vi "HEWH Read Power.vi"(0 "VISA resource name":refnum<visa-resource-name>="WT500", 11 "error in (no error)":errorcluster) -> (3 "PowerClass":T2={"Off"=FALSE, "On"=TRUE, "Logic"=FALSE, "Compressor"=FALSE, "1Heater"=TRUE, "1Heat+Comp"=FALSE, "2Heaters"=FALSE, "2Heat+Comp"=FALSE, "Fault-OverPwr"=FALSE}, 4 "VISA resource name out":refnum<visa-resource-name>="WT500", 6 "PowerData":T1={"Voltage"=236.2, "Current"=17.749, "Power"=4192.0, "WattHours"=0.0}, 15 "error out":errorcluster)   [LabVIEW 2009]
uses:
  PowerClassification.ctl
panel:
  out "CycleCount":dbl
  in  "Local?":bool
  in  "I Range (7: 40A)":u16(ring)=6 items=["AUTO", "500 mA", "1 A", "2 A", "5 A", "10 A", "20 A", "40 A", "S-AUTO", "50 mV", "100 mV", "200 mV", "500 mV", "1 V", "2 V", "5 V", "10 V", "250 mA", "500 mA", "1 A", "2.5 A", "5 A", "10 A", "20 A", "25 mV", "50 mV", "100 mV", "250 mV", "500 mV", "1 V", "2.5 V", "5 V"]
  in  "V Range (8: 1000V)":u16(ring)=6 items=["AUTO", "15", "30", "60", "100", "150", "300", "600", "1000", "7.5", "15", "30", "50", "75", "150", "300", "500"]
  in  "Logic":dbl=5.0
  in  "Fault Limit":dbl=5000.0
  in  "Heating Element":dbl=4300.0
  in  "Compressor":dbl=550.0
  in  "Off Limit":dbl=0.5
  out "Scan Error":bool
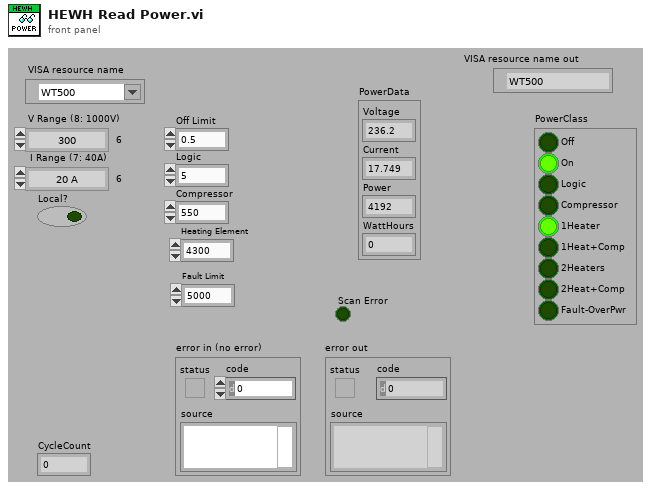
[diagram p1: front panel]
types:
  T1 = cluster{"Voltage":dbl, "Current":dbl, "Power":dbl, "WattHours":dbl}
  T2 = typedef "PowerClassification.ctl" = cluster{"Off":bool, "On":bool, "Logic":bool, "Compressor":bool, "1Heater":bool, "1Heat+Comp":bool, "2Heaters":bool, "2Heat+Comp":bool, "Fault-OverPwr":bool}
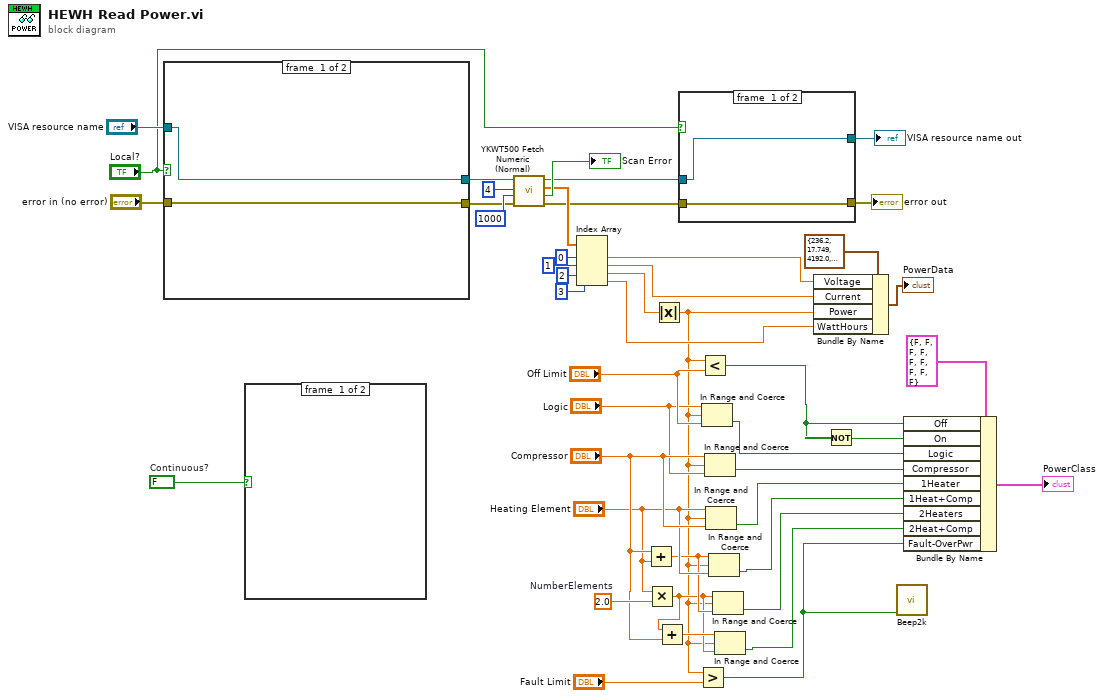
[diagram p0: block diagram]
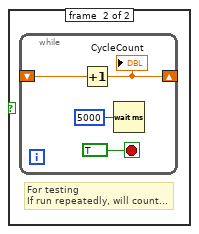
[diagram p2: hidden frame]
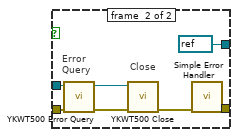
[diagram p3: hidden frame]
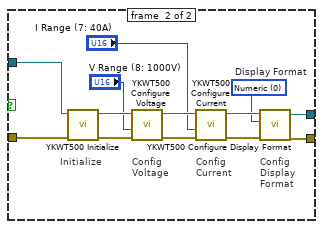
[diagram p4: hidden frame]
diagram:
  w8 = FALSE  # Continuous?
  w36 = 2.0  # NumberElements
  n1 = case shown="True" "Local?" {
    tunnel: "error in (no error)" -> [w46 w51]
    tunnel: "VISA resource name" -> [w47 w50]
    tunnel: [w46 w49] -> w17
    tunnel: [w47 w48] -> w16
    frame #0 {
    }
    frame #1 {
      w52 = u16 0 items=["Numeric", "Wave", "Bar", "Vector", "Trend"]  # Display Format
      # "Config\nDisplay\nFormat"
      # "Config\nCurrent"
      # "Config\nVoltage"
      # "Initialize"
      n2 = call <instrlib>:"YKWT500 Initialize.vi"("error in (no error)"=w51, "VISA resource name"=w50) -> ("error out"=w60:errorcluster, "VISA resource name out"=w58:refnum<visa-resource-name>)  [unwired: 8 in]
      n3 = call <instrlib>:"YKWT500 Configure Voltage.vi"("error in (no error)"=w60, "Voltage Range (8: 1000V)"="V Range (8: 1000V)", "VISA resource name"=w58) -> ("error out"=w59:errorcluster, "VISA resource name out"=w57:refnum<visa-resource-name>)  [unwired: 7 in]
      n4 = call <instrlib>:"YKWT500 Configure Current.vi"("error in (no error)"=w59, "Current Range (7: 40A)"="I Range (7: 40A)", "VISA resource name"=w57) -> ("error out"=w53:errorcluster, "VISA resource name out"=w54:refnum<visa-resource-name>)  [unwired: 7 in]
      n5 = call <instrlib>:"YKWT500 Configure Display Format.vi"("error in (no error)"=w53, "Display Format (0: Numeric)"=w52, "VISA resource name"=w54) -> ("error out"=w49:errorcluster, "VISA resource name out"=w48:refnum<visa-resource-name>)  [unwired: 7 in]
    }
  }
  n6 = case shown="True" w8 {
    frame #0 {
    }
    frame #1 {
      # "For testing\nIf run repeatedly, will count..."
      n7 = while {
        shift-right: [w63] -> _
        shift-left: _ -> [w62]
        stop <- TRUE stop-if-true
        n8 = Increment(x=w62) -> (x+1=w63:dbl)
        "CycleCount" <- w63
        n9 = Wait (ms)(milliseconds to wait=u32 5000) -> ()  [unwired: 1 out]
      }
    }
  }
  n10 = call <instrlib>:"YKWT500 Fetch Numeric (Normal).vi"("error in (no error)"=w17, "Timeout (10000 ms)"=u32 1000, "Number of Item (255)"=4, "VISA resource name"=w16) -> ("error out"=w15:errorcluster, "Scan Error"=→"Scan Error":bool, "Measurement Value"=w42:dbl[], "VISA resource name out"=w13:refnum<visa-resource-name>)  [unwired: 4 in]
  n11 = Index Array(array=w42, index #1=0 ("index"), index #2=1 ("index"), index #3=2 ("index"), index #4=3 ("index")) -> (element #1=w1:dbl, element #2=w2:dbl, element #3=w38:dbl, element #4=w4:dbl)
  n12 = Add(x="Compressor", y="Heating Element") -> (x+y=w21:dbl)
  n13 = Multiply(x="Heating Element", y=w36) -> (x*y=w20:dbl)
  n14 = Absolute Value(x=w38) -> (abs(x)=w3:dbl)
  n15 = Add(x=w20, y="Compressor") -> (x+y=w34:dbl)
  n16 = case shown="True" "Local?" {
    tunnel: w15 -> [w65 w70]
    tunnel: [w65 w69] -> w14
    tunnel: w13 -> [w66 w68]
    tunnel: [w66 refnum<visa-resource-name> refnum ("VISA resource name out")] -> w11
    frame #0 {
    }
    frame #1 {
      # "Error\nQuery"
      # "Close"
      n17 = call <instrlib>:"YKWT500 Error Query.vi"("error in (no error)"=w70, "VISA resource name"=w68) -> ("error out"=w72:errorcluster, "VISA resource name out"=w71:refnum<visa-resource-name>)  [unwired: 6 in, 2 out]
      n18 = call <instrlib>:"YKWT500 Close.vi"("error in (no error)"=w72, "VISA resource name"=w71) -> ("error out"=w73:errorcluster)  [unwired: 9 in]
      n19 = call <vilib>:"Simple Error Handler.vi"("error in (no error)"=w73) -> ("error out"=w69:errorcluster)  [unwired: 4 in, 4 out]
    }
  }
  "error out" <- w14
  "VISA resource name out" <- w11
  n20 = Greater?(x=w3, y="Fault Limit") -> (0:w9:bool)
  n21 = Less?(x=w3, y="Off Limit") -> (x < y?=w31:bool)
  n22 = In Range and Coerce(upper limit="Logic", x=w3, lower limit="Off Limit") -> (In Range?=w29:bool)  [unwired: 1 out]
  n23 = In Range and Coerce(upper limit="Compressor", x=w3, lower limit="Logic") -> (In Range?=w28:bool)  [unwired: 1 out]
  n24 = In Range and Coerce(upper limit="Heating Element", x=w3, lower limit="Compressor") -> (In Range?=w27:bool)  [unwired: 1 out]
  n25 = In Range and Coerce(upper limit=w21, x=w3, lower limit="Heating Element") -> (In Range?=w26:bool)  [unwired: 1 out]
  n26 = In Range and Coerce(upper limit=w20, x=w3, lower limit=w21) -> (In Range?=w25:bool)  [unwired: 1 out]
  n27 = In Range and Coerce(upper limit=w34, x=w3, lower limit=w20) -> (In Range?=w24:bool)  [unwired: 1 out]
  n28 = Bundle By Name(cluster=T1 {"Voltage"=236.2, "Current"=17.749, "Power"=4192.0, "WattHours"=0.0} ("PowerData 3"), "Voltage"=w1, "Current"=w2, "Power"=w3, "WattHours"=w4) -> (→"PowerData":T1)
  n29 = Not(x=w31) -> (.not. x?=w32:bool)
  n30 = call "Beep2k.vi"("Beep?"=w9) -> ()  [unwired: 11 in]
  n31 = Bundle By Name(cluster=T2 {"Off"=FALSE, "On"=FALSE, "Logic"=FALSE, "Compressor"=FALSE, "1Heater"=FALSE, "1Heat+Comp"=FALSE, "2Heaters"=FALSE, "2Heat+Comp"=FALSE, "Fault-OverPwr"=FALSE} ("PowerClass 2"), "Off"=w31, "On"=w32, "Logic"=w29, "Compressor"=w28, "1Heater"=w27, "1Heat+Comp"=w26, "2Heaters"=w25, "2Heat+Comp"=w24, "Fault-OverPwr"=w9) -> (→"PowerClass":T2)
